vi "Update Active Filters.vi"(8 "error in":errorcluster, 11 "Configuration":T1={"Data Tree Ref"=refnum, "FP Ref"=refnum, "Column Data Type"=[], "Search Clones Up To"=0, "SortOptions"={"Col.pri"=0, "RevDir.pri"=FALSE, "Col.sec"=0, "RevDir.sec"=FALSE}, "Group/Flat (0:group)"=FALSE, "CollapsedNodes"=[], "Show/Hide Cols"=[], "Filtered Paths"=[], "View"=enum."Group By Library", "File Extension Filters"=[], "Filter Global VIs"=FALSE, "Shared"=refnum, "Active Filters"=refnum, "Refresh Rate (ms)"=2000}) -> (0 "error out":errorcluster)   [LabVIEW 2013, in "LVTM.lvlib"]
uses:
  LVTM.lvlib
  Controls_LVTM/LVTM_Config_Info.ctl
  Controls_LVTM/View.ctl
  Controls_LVTM/SharedDataDVR.ctl
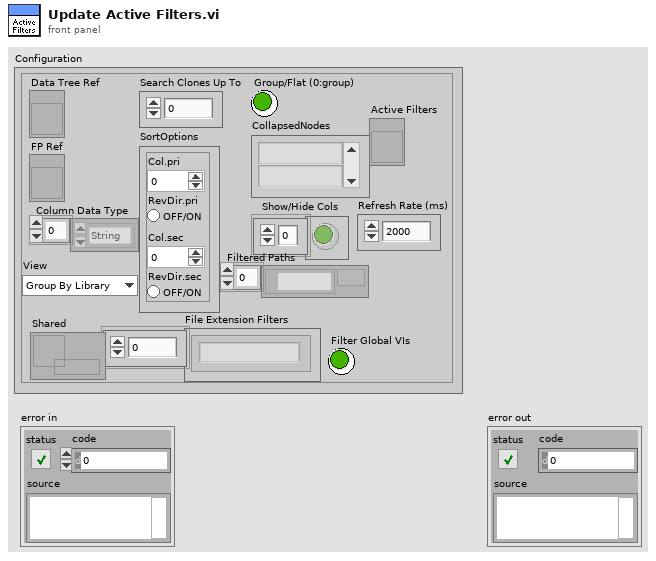
[diagram p1: front panel]
types:
  T1 = typedef "LVTM.lvlib/LVTM_Config_Info.ctl" = cluster{"Data Tree Ref":refnum<vi>, "FP Ref":refnum<vi>, "Column Data Type":enum16{"String", "Numeric"}[], "Search Clones Up To":i32, "SortOptions":cluster{"Col.pri":i32, "RevDir.pri":bool, "Col.sec":i32, "RevDir.sec":bool}, "Group/Flat (0:group)":bool, "CollapsedNodes":string[], "Show/Hide Cols":bool[], "Filtered Paths":path[], "View":T2, "File Extension Filters":string[], "Filter Global VIs":bool, "Shared":refnum<data-value>, "Active Filters":refnum<vi>, "Refresh Rate (ms)":i32}
  T2 = typedef "LVTM.lvlib/View.ctl" = enum16{"Group By Library", "Group By Folder", "Flat List"}
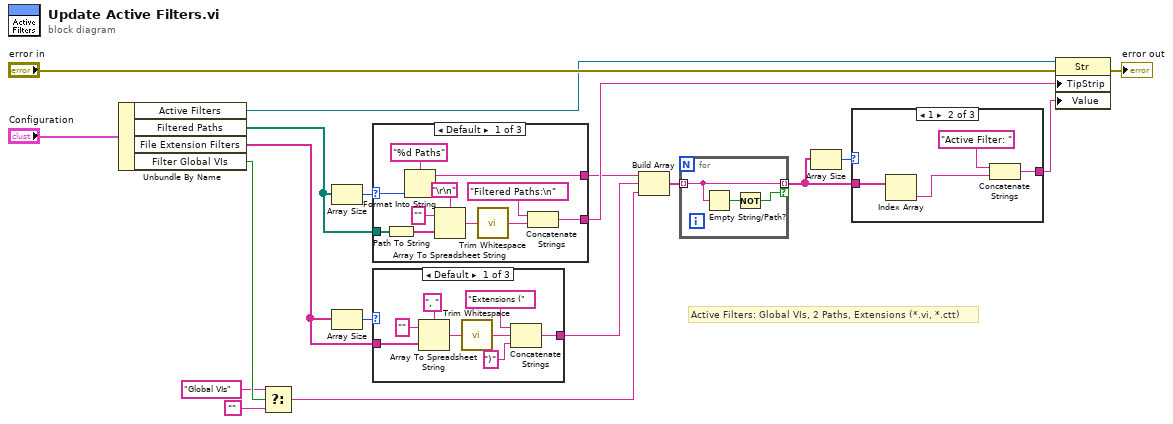
[diagram p0: block diagram]
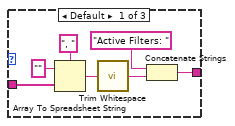
[diagram p2: hidden frame]
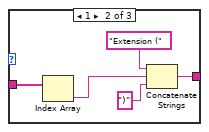
[diagram p4: hidden frame]
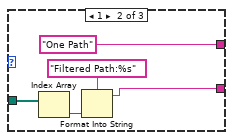
[diagram p6: hidden frame]
diagram:
  # "Active Filters: Global VIs, 2 Paths, Extensions (*.vi, *.ctt)"
  n1 = Unbundle By Name("Configuration") -> ("Active Filters"=w17:refnum<vi>, "Filtered Paths"=w9:path[], "File Extension Filters"=w10:string[], "Filter Global VIs"=w15:bool)
  n2 = Select(t="Global VIs", s=w15, f="") -> (s? t:f=w5:string)
  n3 = Array Size(array=w9) -> (size(s)=w12:i32)
  n4 = Array Size(array=w10) -> (size(s)=w11:i32)
  n5 = case shown="Default" w12 {
    selector: w12 -> [w30 _ _]
    tunnel: [w28 "One Path" _] -> w7
    tunnel: w9 -> [w27 w34 _]
    tunnel: [w20 w31 _] -> w8
    frame Default {
      n6 = Path To String(path=w27) -> (string=w23:string[])
      n7 = Format Into String(format string="%d Paths", w30) -> (resulting string=w28:string)  [unwired: 2 in, 1 out]
      n8 = Array To Spreadsheet String(delimiter (Tab)="\r\n", array=w23, 3:"" ("format string")) -> (spreadsheet string=w26:string)
      n9 = call <vilib>:"Trim Whitespace.vi"("string"=w26) -> ("trimmed string"=w21:string)  [unwired: 1 in]
      n10 = Concatenate Strings("Filtered Paths:\n" ("format string"), w21) -> (w20:string)
    }
    frame 1 {
      n11 = Index Array(array=w34) -> (element=w33:path)  [unwired: 1 in]
      n12 = Format Into String(format string="Filtered Path:%s", w33) -> (resulting string=w31:string)  [unwired: 2 in, 1 out]
    }
    frame 0 {
    }
  }
  n13 = case shown="Default" w11 {
    tunnel: w10 -> [w41 w45 _]
    tunnel: [w36 w46 _] -> w6
    frame Default {
      n14 = Array To Spreadsheet String(delimiter (Tab)=", ", array=w41, 3:"" ("format string")) -> (spreadsheet string=w40:string)
      n15 = call <vilib>:"Trim Whitespace.vi"("string"=w40) -> ("trimmed string"=w39:string)  [unwired: 1 in]
      n16 = Concatenate Strings("Extensions (" ("format string"), w39, ")" ("format string")) -> (w36:string)
    }
    frame 1 {
      n17 = Index Array(array=w45) -> (element=w44:string)  [unwired: 1 in]
      n18 = Concatenate Strings("Extension (" ("format string"), w44, ")" ("format string")) -> (w46:string)
    }
    frame 0 {
    }
  }
  n19 = Build Array(w7, w6, w5) -> (w4:string[])
  n20 = for {
    tunnel: w4 -> [w51] mode=indexing
    tunnel: [w51] -> w2 mode=indexing if=w49
    n21 = Empty String/Path?(string/path=w51) -> (empty?=w50:bool)
    n22 = Not(x=w50) -> (.not. x?=w49:bool)
  }
  n23 = Array Size(array=w2) -> (size(s)=w3:i32)
  n24 = case shown="1" w3 {
    tunnel: w2 -> [w56 w60 _]
    tunnel: [w52 w61 _] -> w1
    frame Default {
      n25 = Array To Spreadsheet String(delimiter (Tab)=", ", array=w56, 3:"" ("format string")) -> (spreadsheet string=w55:string)
      n26 = call <vilib>:"Trim Whitespace.vi"("string"=w55) -> ("trimmed string"=w54:string)  [unwired: 1 in]
      n27 = Concatenate Strings("Active Filters: " ("format string"), w54) -> (w52:string)
    }
    frame 1 {
      n28 = Index Array(array=w60) -> (element=w59:string)  [unwired: 1 in]
      n29 = Concatenate Strings("Active Filter: " ("format string"), w59) -> (w61:string)
    }
    frame 0 {
    }
  }
  n30 = property class="Str"(reference=w17, error in="error in", "TipStrip"=w8, "Value"=w1) -> (error out=→"error out":errorcluster)  [unwired: 1 out]
